vi "Remove Item from ListBox.vi"(8 "error in (no error)":errorcluster, 11 "MulticolumnListbox in":refnum<vi>) -> (0 "error out":errorcluster)   [LabVIEW 2015, in "Diagnostics Addon System Explorer.lvlib"]
uses:
  Diagnostics Addon System Explorer.lvlib
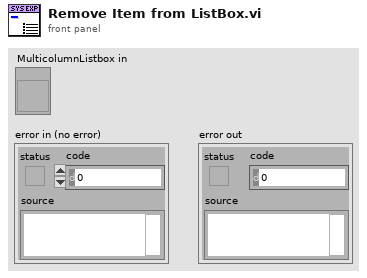
[diagram p1: front panel]
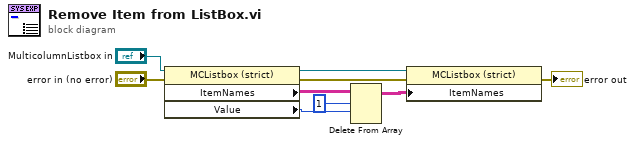
[diagram p0: block diagram]
diagram:
  n1 = property class="MCListbox (strict)"(reference="MulticolumnListbox in", error in="error in (no error)") -> (reference out=w2:refnum<vi>, error out=w6:errorcluster, "ItemNames"=w3:string[][], "Value"=w9:i32)
  n2 = Delete From Array(array=w3, length=1, index (row)=w9) -> (array with subset deleted=w4:string[][])  [unwired: 1 in, 1 out]
  n3 = property class="MCListbox (strict)"(reference=w2, error in=w6, "ItemNames"=w4) -> (error out=→"error out":errorcluster)  [unwired: 1 out]
